vi "Edit Config.vi"(8 "error in (no error)":errorcluster, 11 "Serial in":refnum<class "Serial.lvclass">) -> (0 "error out":errorcluster, 3 "Serial out":refnum<class "Serial.lvclass">)   [LabVIEW 2024, in "Serial.lvclass"]
doc: "Serial.lvclass:Edit Config.vi\n\nThis VI is used to edit the Serial configuration parameters.\n\nInstrument Communication Module Version 1.0\nJuly, 2017 Original Code Consulting David Thomson\n www.originalcode.com"
uses:
  Serial.lvclass
  Serial Config.ctl
  ICM Class Editor State.ctl
  ICM Editor Command.ctl
  Serial.lvclass/Serial.ctl
panel:
  out "Serial Ports":i32[](array[numeric])
  in  "Check":bool
  in  "Flash Save":bool
  in  "Save":bool
  in  "Revert":bool
  in  "Serial Config":T1={"Port"=4, "Baud Rate"=115200, "Data Bits"=8, "Parity"=enum."None", "Stop Bits"=10, "Flow Control"=0, "Char/Record"=0, "Termination String"="", "ms Wait"=1000, "Time-out (1000ms)"=1000, "Clear Buffer on Open?"=FALSE} {"Flow Control" items=["None", "XON/XOFF", "RTS/CTS", "XON/XOFF & RTS/CTS", "DTR/DSR", "XON/XOFF & DTR/DSR"]; "Stop Bits" items=["1.0"=10, "1.5"=15, "2.0"=20]; "Data Bits" min=5 max=8 step=1}
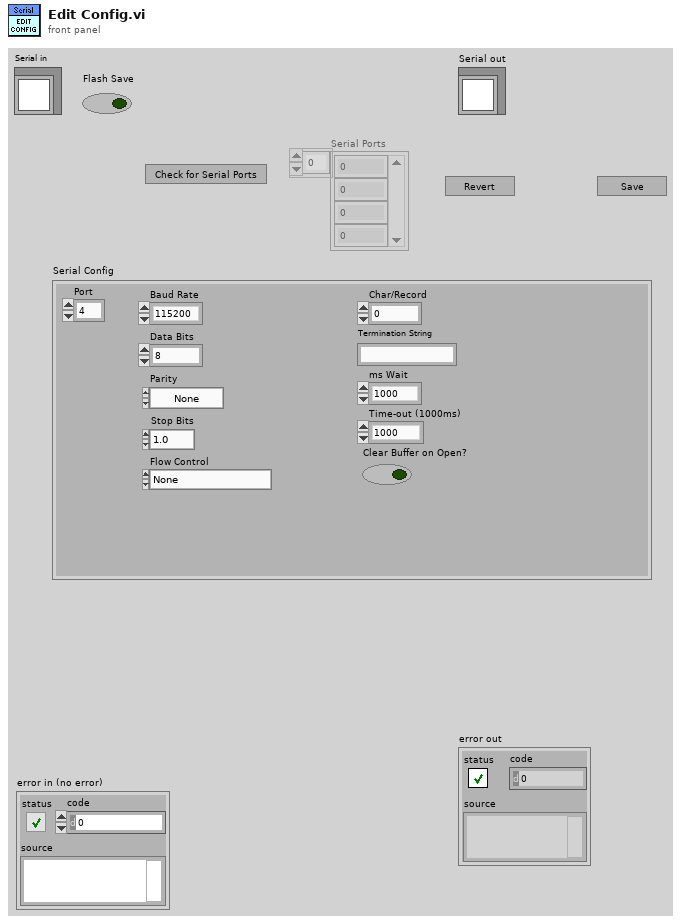
[diagram p1: front panel]
types:
  T1 = typedef "Serial.lvclass/Serial Config.ctl" = cluster{"Port":i32, "Baud Rate":u32, "Data Bits":u16, "Parity":enum16{"None", "Odd", "Even", "Mark", "Space"}, "Stop Bits":u16, "Flow Control":u16, "Char/Record":i32, "Termination String":string, "ms Wait":u32, "Time-out (1000ms)":u32, "Clear Buffer on Open?":bool}
  T2 = typedef "ICM Editor Command.ctl" = enum16{"No-op", "Exit"}
  T3 = typedef "ICM Class Editor State.ctl" = enum16{"Init", "Wait", "Write", "Read", "Display", "Set Flashing", "Error", "Stop"}
  T4 = enum8{"Enabled", "Disabled", "Disabled and Grayed Out"}
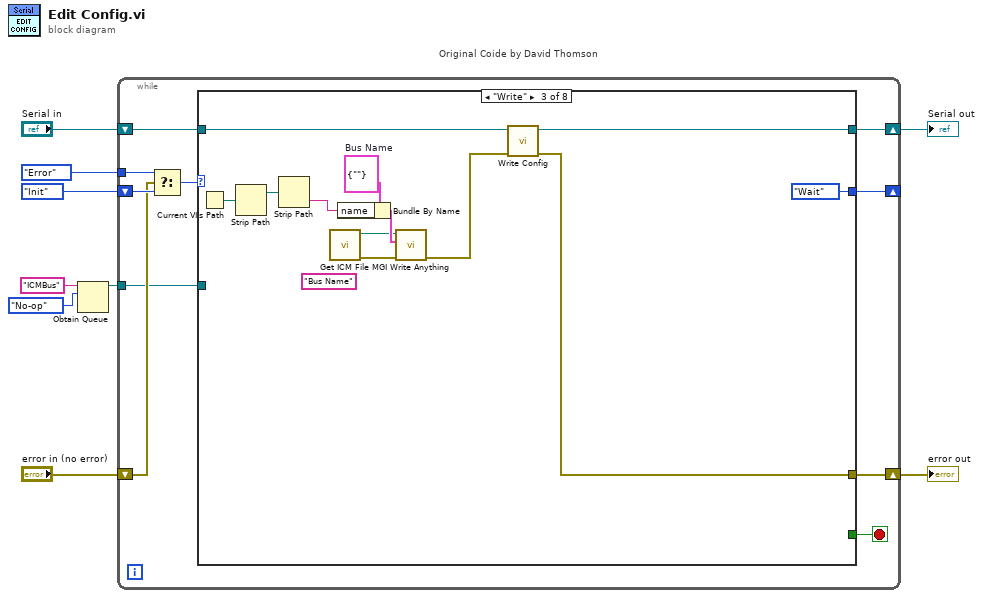
[diagram p0: block diagram]
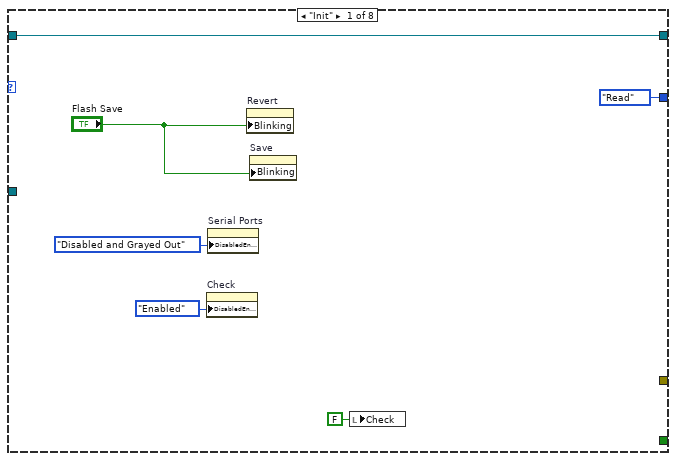
[diagram p2: hidden frame]
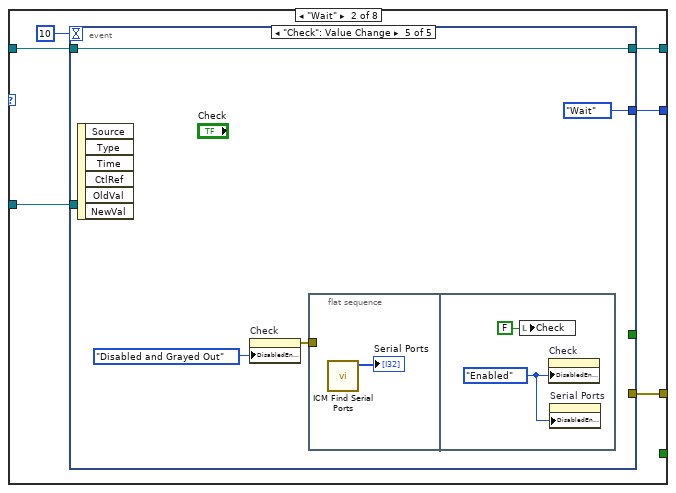
[diagram p3: hidden frame]
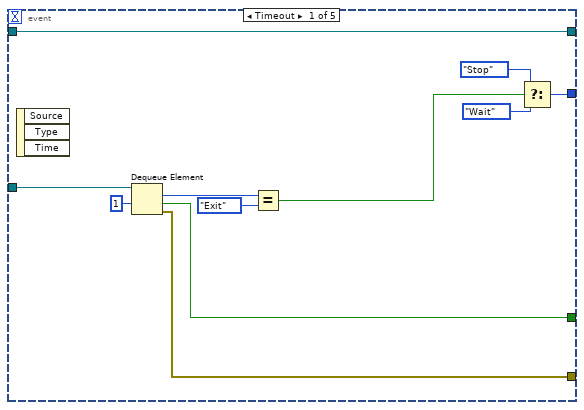
[diagram p4: hidden frame]
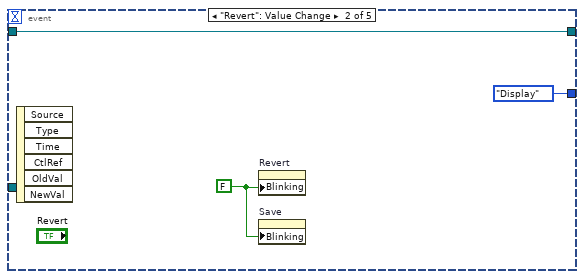
[diagram p5: hidden frame]
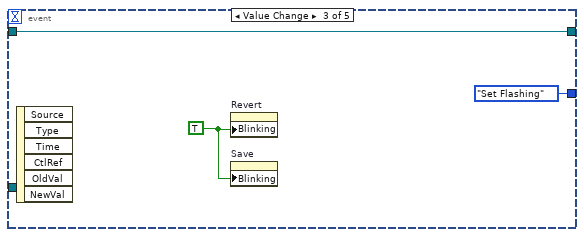
[diagram p6: hidden frame]
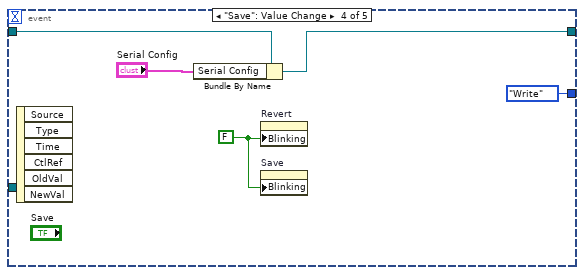
[diagram p7: hidden frame]
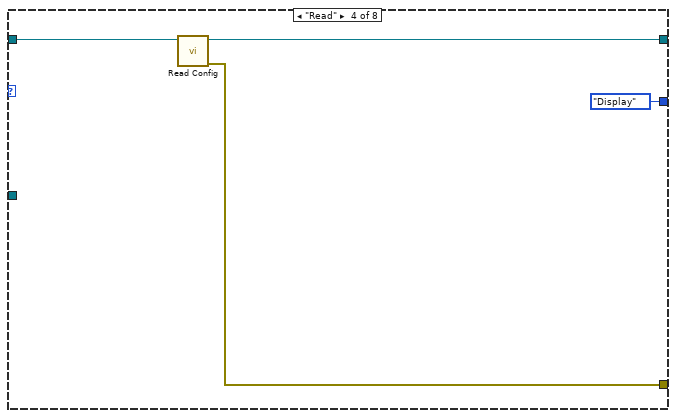
[diagram p8: hidden frame]
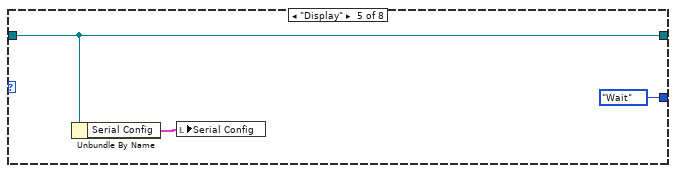
[diagram p9: hidden frame]
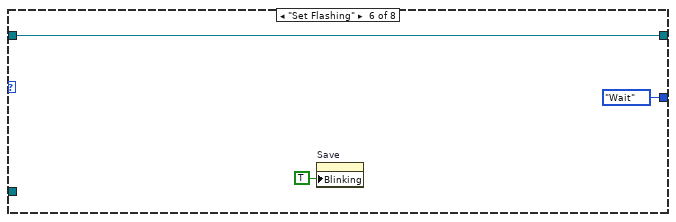
[diagram p10: hidden frame]
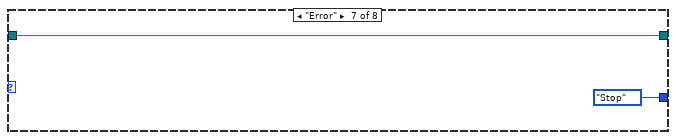
[diagram p11: hidden frame]
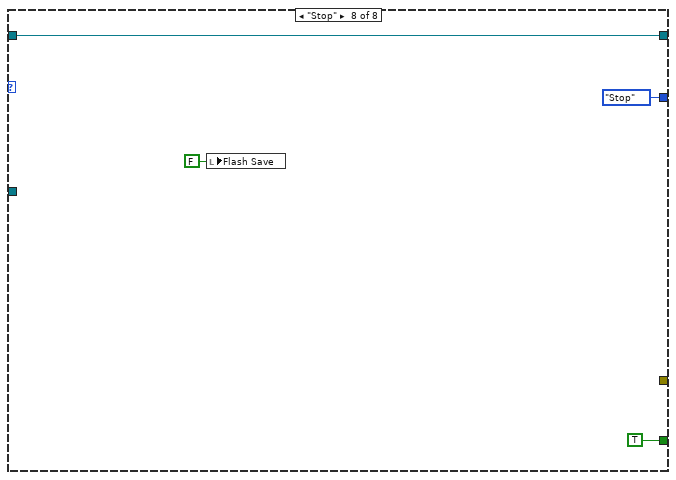
[diagram p12: hidden frame]
diagram:
  n1 = Obtain Queue(name (unnamed)="ICMBus", element data type=ICM_Editor_Command."No-op" ("Editor Command")) -> (queue out=w1:refnum<queue>)  [unwired: 3 in, 2 out]
  n2 = while "Original Coide by David Thomson" {
    shift-right: [w19] -> w8
    shift-left: "Serial in" -> [w18]
    shift-right: [w12] -> _
    shift-left: ICM_Class_Editor_State."Init" ("Config State") -> [w16]
    shift-right: [w11] -> w6
    shift-left: "error in (no error)" -> [w14]
    tunnel: ICM_Class_Editor_State."Error" ("Config State") -> [w13]
    tunnel: w1 -> [w10]
    stop <- w17 stop-if-true
    n3 = Select(t=w13, s=w14, f=w16) -> (s? t:f=w15:T3)
    n4 = case shown="\"Write\"" w15 {
      tunnel: [w24 w29 w70 w74 w79 w82 w84 w88] -> w19
      tunnel: w18 -> [w24 w28 w71 w76 w79 w82 w84 w88]
      tunnel: [_ _ _ _ _ _ _ TRUE] -> w17
      tunnel: [ICM_Class_Editor_State."Read" ("Config State") w30 ICM_Class_Editor_State."Wait" ("Config State") ICM_Class_Editor_State."Display" ("Config State") ICM_Class_Editor_State."Wait" ("Config State") ICM_Class_Editor_State."Wait" ("Config State") ICM_Class_Editor_State."Stop" ("Config State") ICM_Class_Editor_State."Stop" ("Config State")] -> w12
      tunnel: [_ w26 w69 w75 _ _ _ _] -> w11
      tunnel: w10 -> [_ w27 _ _ _ _ _ _]
      frame "Init" {
        n5 = property on="Check" class="Bool (strict)"("DisabledEnum"=T4."Enabled" ("Disabled")) -> ()  [unwired: 2 in, 2 out]
        n6 = property on="Serial Ports" class="Arr (strict)"("DisabledEnum"=T4."Disabled and Grayed Out" ("Disabled")) -> ()  [unwired: 2 in, 2 out]
        n7 = property on="Revert" class="Bool"("Blinking"="Flash Save") -> ()  [unwired: 2 in, 2 out]
        n8 = property on="Save" class="Bool"("Blinking"="Flash Save") -> ()  [unwired: 2 in, 2 out]
        n9 = local write "Check"(FALSE ("Check")) -> ()
      }
      frame "Wait" {
        n10 = event shown="[4] \"Check\": Value Change" {
          selector: _ -> [_ _ _ _ _]
          dyn-events: _ -> [_ _ _ _ _]
          timeout: 10 -> [_ _ _ _ _]
          tunnel: [w39 ICM_Class_Editor_State."Display" ("Config State") ICM_Class_Editor_State."Set Flashing" ("Config State") ICM_Class_Editor_State."Write" ("Config State") ICM_Class_Editor_State."Wait" ("Config State")] -> w30
          tunnel: [w42 w44 w48 w50 w57] -> w29
          tunnel: w28 -> [w42 w44 w48 w51 w57]
          tunnel: w27 -> [w41 _ _ _ _]
          tunnel: [w33 _ _ _ _] -> w26
          tunnel: [w32 _ _ _ _] -> _
          event Timeout {
            n11 = event-data() -> ()  [unwired: 1 in, 3 out]
            n12 = Dequeue Element(queue=w41, timeout in ms (-1)=1) -> (element=w38:T2, timed out?=w32:bool, error out=w33:errorcluster)  [unwired: 1 in, 1 out]
            n13 = Equal?(x=w38, y=ICM_Editor_Command."Exit") -> (x = y?=w36:bool)
            n14 = Select(t=ICM_Class_Editor_State."Stop" ("Config State"), s=w36, f=ICM_Class_Editor_State."Wait" ("Config State")) -> (s? t:f=w39:T3)
          }
          event "Revert": Value Change {
            w43 = FALSE ("Blinking")
            n15 = event-data() -> ()  [unwired: 1 in, 6 out]
            n16 = property on="Revert" class="Bool"("Blinking"=w43) -> ()  [unwired: 2 in, 2 out]
            n17 = property on="Save" class="Bool"("Blinking"=w43) -> ()  [unwired: 2 in, 2 out]
          }
          event Value Change {
            w46 = TRUE ("Blinking")
            n18 = event-data() -> ()  [unwired: 1 in, 6 out]
            n19 = property on="Revert" class="Bool"("Blinking"=w46) -> ()  [unwired: 2 in, 2 out]
            n20 = property on="Save" class="Bool"("Blinking"=w46) -> ()  [unwired: 2 in, 2 out]
          }
          event "Save": Value Change {
            w49 = FALSE ("Blinking")
            n21 = event-data() -> ()  [unwired: 1 in, 6 out]
            n22 = Bundle By Name(cluster=w51, "Serial Config"="Serial Config") -> (w50:refnum<class "Serial.lvclass">)
            n23 = property on="Revert" class="Bool"("Blinking"=w49) -> ()  [unwired: 2 in, 2 out]
            n24 = property on="Save" class="Bool"("Blinking"=w49) -> ()  [unwired: 2 in, 2 out]
          }
          event "Check": Value Change {
            n25 = event-data() -> ()  [unwired: 1 in, 6 out]
            n26 = property on="Check" class="Bool (strict)"("DisabledEnum"=T4."Disabled and Grayed Out" ("Disabled")) -> (error out=w55:errorcluster)  [unwired: 2 in, 1 out]
            n27 = flat-sequence {
              tunnel: w55 -> [_]
              frame #0 {
                n28 = call "ICM Find Serial Ports.vi"() -> ("Serial Ports"=→"Serial Ports":i32[])  [unwired: 11 in]
              }
              frame #1 {
                w59 = T4."Enabled" ("Disabled")
                n29 = local write "Check"(FALSE ("Check")) -> ()
                n30 = property on="Check" class="Bool (strict)"("DisabledEnum"=w59) -> ()  [unwired: 2 in, 2 out]
                n31 = property on="Serial Ports" class="Arr (strict)"("DisabledEnum"=w59) -> ()  [unwired: 2 in, 2 out]
              }
            }
          }
        }
      }
      frame "Write" {
        w65 = cluster{"name":string} {"name"=""}  # Bus Name
        (unwired) "Bus Name" ("Section Name (Name of \"Anything\")")
        n32 = Current VI's Path() -> (path=w68:path)
        n33 = Strip Path(path=w68) -> (stripped path=w67:path)  [unwired: 1 out]
        n34 = Strip Path(path=w67) -> (name=w64:string)  [unwired: 1 out]
        n35 = call "Get ICM File.vi"() -> ("error out"=w66:errorcluster, "ICM File"=w61:path)  [unwired: 10 in]
        n36 = Bundle By Name(cluster=w65, "name"=w64) -> (w63:cluster{"name":string})
        n37 = call "MGI Write Anything.vi"("Error In"=w66, "Anything"=w63, "Path (dialog)"=w61) -> ("Error Out"=w62:errorcluster)  [unwired: 6 in, 2 out]
        n38 = call-dynamic "Write Config.vi"("error in (no error)"=w62, "Serial in"=w71) -> ("error out"=w69:errorcluster, "Serial out"=w70:refnum<class "Serial.lvclass">)  [unwired: 8 in]
      }
      frame "Read" {
        n39 = call-dynamic "Read Config.vi"("Serial in"=w76) -> ("error out"=w75:errorcluster, "Serial out"=w74:refnum<class "Serial.lvclass">)  [unwired: 9 in]
      }
      frame "Display" {
        n40 = Unbundle By Name(w79) -> ("Serial Config"=w78:T1)
        n41 = local write "Serial Config"(w78) -> ()
      }
      frame "Set Flashing" {
        n42 = property on="Save" class="Bool"("Blinking"=TRUE) -> ()  [unwired: 2 in, 2 out]
      }
      frame "Error" {
      }
      frame "Stop" {
        n43 = local write "Flash Save"(FALSE ("Flash Save")) -> ()
      }
    }
  }
  "error out" <- w6
  "Serial out" <- w8
